vi "2-Read-SRC-varid.vi"(6 "err in":errorcluster, 9 "code src":string, 11 "tdms in":refnum<k34>) -> (1 "varid":T1, 3 "tdms out":refnum<k34>, 4 "error out":errorcluster caption="err out", 5 "txt_desc_TDMS":string[](array[string]), 7 "ent_desc_TDMS":string[](array[string]))   [LabVIEW 2010, in "lv_04.lvlib"]
uses:
  lv_04.lvlib
  commandes/cSTA_varid.ctl
  commandes/c_TDMS_ch_variable.ctl
  commandes/c_TDMS_ch_donnees.ctl
  commandes/c0-var-n.ctl
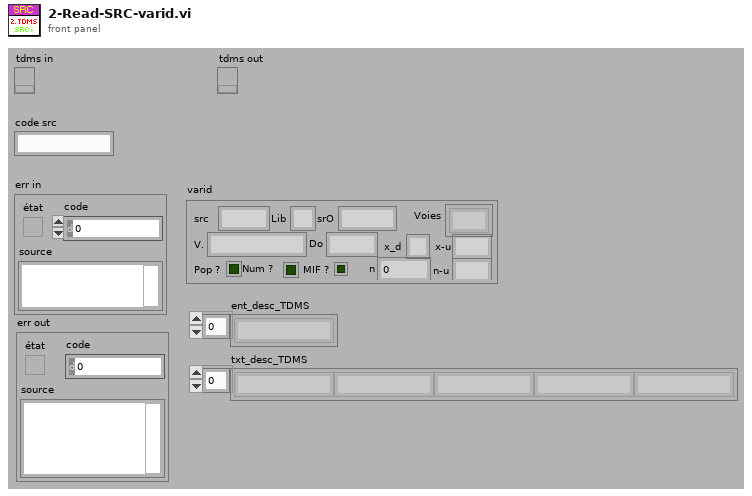
[diagram p1: front panel]
types:
  T1 = typedef "lv_04.lvlib/cSTA_varid.ctl" = cluster{"src":string, "Lib":string, "srO":string, "V.":T2, "Voies":string[], "Do":T3, "n":T4, "Num ?":bool, "Pop ?":bool, "x_d":string, "x-u":string, "n-u":string, "MIF ?":bool}
  T2 = typedef "lv_04.lvlib/c_TDMS_ch_variable.ctl" = string
  T3 = typedef "lv_04.lvlib/c_TDMS_ch_donnees.ctl" = string
  T4 = typedef "lv_04.lvlib/c0-var-n.ctl" = i32
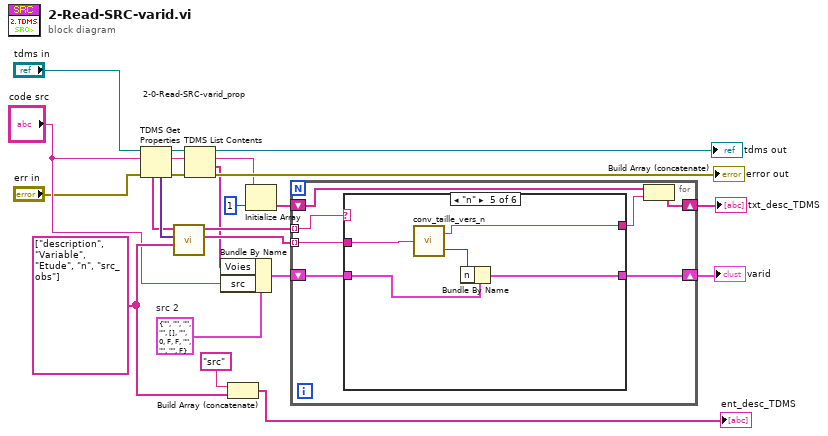
[diagram p0: block diagram]
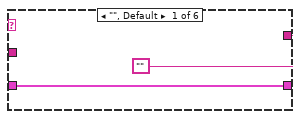
[diagram p2: hidden frame]
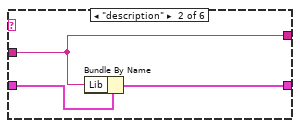
[diagram p3: hidden frame]
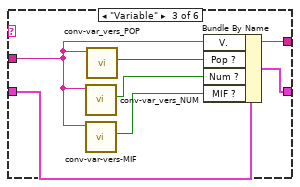
[diagram p4: hidden frame]
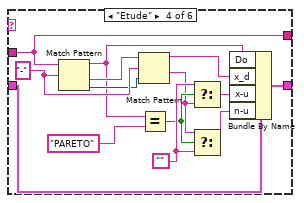
[diagram p5: hidden frame]
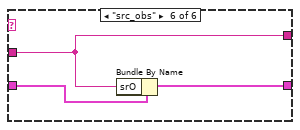
[diagram p6: hidden frame]
diagram:
  w5 = T1 {"src"="", "Lib"="", "srO"="", "V."="", "Voies"=[], "Do"="", "n"=0, "Num ?"=FALSE, "Pop ?"=FALSE, "x_d"="", "x-u"="", "n-u"="", "MIF ?"=FALSE}  # src 2
  w22 = string[] ["description", "Variable", "Etude", "n", "src_obs"]
  n1 = TDMS Get Properties ("TDMS - Obtenir des propriétés")(8:"err in", 10:"code src", 11:"tdms in") -> (0:w7:errorcluster, 2:w3:string, 3:w18:refnum<k34>, 4:w10:variant[], 6:w9:string[])  [unwired: 3 in, 1 out]
  n2 = call "2-0-Read-SRC-varid_prop.vi"("prop_src (entrée)"=w22, "valeurs prop (variant)"=w10, "liste_prop"=w9) -> ("valeurs prop_src"=w12:string[], "prop_src (sortie)"=w11:string[])  [unwired: 3 in]
  n3 = TDMS List Contents ("TDMS - Répertorier le contenu")(4:w7, 6:w3, 7:w18) -> (0:→"error out":errorcluster, 1:w2:string[], 2:w4:string, 3:→"tdms out":refnum<k34>)
  n4 = Bundle By Name(cluster=w5, "Voies"=w2, "src"="code src") -> (w13:T1)
  n5 = Build Array (concatenate)("src", w22) -> (→"ent_desc_TDMS":string[])
  n6 = Initialize Array(w4, 1 ("taille de la dimension")) -> (w15:string[])
  n7 = for {
    tunnel: w11 -> [w30] mode=indexing
    tunnel: w12 -> [w28] mode=indexing
    shift-right: [w24] -> w1
    shift-left: w13 -> [w29]
    shift-right: [w26] -> w16
    shift-left: w15 -> [w27]
    n8 = case shown="\"n\"" w30 {
      tunnel: w29 -> [w32 w35 w40 w55 w58 w62]
      tunnel: [w32 w34 w39 w54 w56 w63] -> w24
      tunnel: w28 -> [_ w33 w37 w50 w59 w61]
      tunnel: ["" w33 w37 w50 w60 w61] -> w25
      frame "", Default {
      }
      frame "description" {
        n9 = Bundle By Name(cluster=w35, "Lib"=w33) -> (w34:T1)
      }
      frame "Variable" {
        n10 = call "conv-var_vers_NUM.vi"("Variable"=w37) -> ("Num ?"=w38:bool)  [unwired: 4 in, 2 out]
        n11 = call "conv-var-vers-MIF.vi"("Variable"=w37) -> ("MIF ?"=w36:bool)  [unwired: 4 in, 2 out]
        n12 = call "conv-var_vers_POP.vi"("Variable"=w37) -> ("Pop ?"=w41:bool)  [unwired: 4 in, 2 out]
        n13 = Bundle By Name(cluster=w40, "V."=w37, "Pop ?"=w41, "Num ?"=w38, "MIF ?"=w36) -> (w39:T1)
      }
      frame "Etude" {
        w45 = ""
        w52 = "-" ("expression régulière")
        n14 = Match Pattern(string=w50, regular expression=w52) -> (before substring=w47:string, after substring=w53:string, offset past match=w51:i32)  [unwired: 1 in, 1 out]
        n15 = Match Pattern(string=w53, regular expression=w52, offset (0)=w51) -> (before substring=w49:string, after substring=w43:string)  [unwired: 2 out]
        n16 = Equal?(x=w47, y="PARETO") -> (x = y?=w44:bool)
        n17 = Select(t=w45, s=w44, f=w43) -> (s? t:f=w42:string)
        n18 = Select(t=w43, s=w44, f=w45) -> (s? t:f=w48:string)
        n19 = Bundle By Name(cluster=w55, "Do"=w47, "x_d"=w49, "x-u"=w42, "n-u"=w48) -> (w54:T1)
      }
      frame "n" {
        n20 = call "conv_taille_vers_n.vi"("taille"=w59) -> ("val_effectif"=w57:i32, "ch_effectif"=w60:string)
        n21 = Bundle By Name(cluster=w58, "n"=w57) -> (w56:T1)
      }
      frame "src_obs" {
        n22 = Bundle By Name(cluster=w62, "srO"=w61) -> (w63:T1)
      }
    }
    n23 = Build Array (concatenate)(w27, w25) -> (w26:string[])
  }
  "txt_desc_TDMS" <- w16
  "varid" <- w1
